vi "Open Waveform File Plot.vi"(8 "error in (no error)":errorcluster, 10 "File Path Control":path, 11 "Measure Controller in":refnum<class "Measure Controller.lvclass">) -> (0 "error out":errorcluster, 3 "Measure Controller out":refnum<class "Measure Controller.lvclass">)   [LabVIEW 2015, in "Measure Controller.lvclass"]
uses:
  Measure Controller.lvclass
  Plots/Waveform Plot/Waveform Plot.lvclass
  Plots/Plot/Plot.lvclass/Plot.ctl
  <vilib>/ActorFramework/Message Enqueuer/Message Enqueuer.lvclass/Message Enqueuer.ctl
  Plots/Plot/Write File-group-channel.vi
  <vilib>/ActorFramework/Message Enqueuer/Enqueue.vi
  <vilib>/ActorFramework/Message Priority Queue/Priority Enqueue.vi
  Measure Object Messages/Open Front Panel Msg/Open Front Panel Msg.lvclass
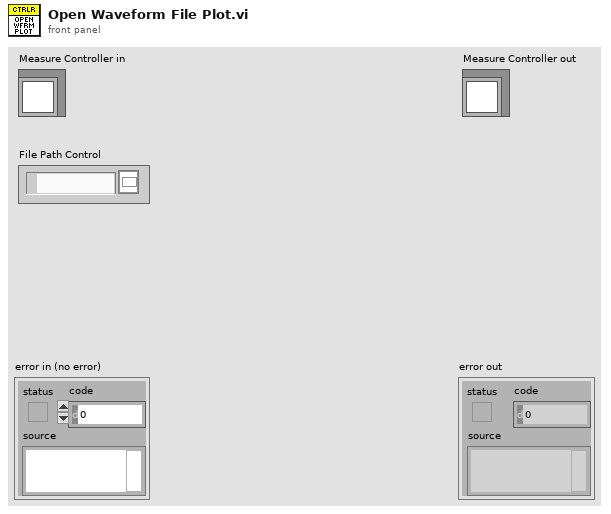
[diagram p1: front panel]
types:
  T1 = cluster{"File Path Control":path, "Group":string, "Channel":string, "Abbreviated":string}
  T2 = cluster{"File Path Control":path, "Group":string, "Channel":string, "Abbreviated":string}[]
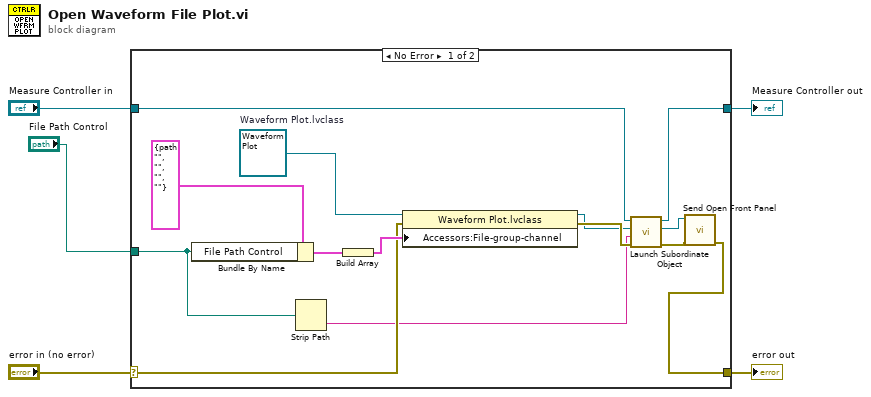
[diagram p0: block diagram]
diagram:
  n1 = case shown="No Error" "error in (no error)" {
    selector: "error in (no error)" -> [w15 w21]
    tunnel: [w6 w21] -> w4
    tunnel: [w13 w20] -> w2
    tunnel: "Measure Controller in" -> [w14 w20]
    tunnel: "File Path Control" -> [w10 _]
    frame No Error {
      w19 = refnum<class "Waveform Plot.lvclass"> refnum  # Waveform Plot.lvclass
      n2 = Bundle By Name(cluster=T1 {"File Path Control"=path "", "Group"="", "Channel"="", "Abbreviated"=""} ("Cluster"), "File Path Control"=w10) -> (w17:T1)
      n3 = Strip Path(path=w10) -> (name=w9:string)  [unwired: 1 out]
      n4 = Build Array(w17) -> (w16:T2)
      n5 = property class="Waveform Plot.lvclass"(reference=w19, error in=w15, "Accessors:File-group-channel"=w16) -> (reference out=w11:refnum<class "Waveform Plot.lvclass">, error out=w12:errorcluster)
      n6 = call-dynamic "Launch Subordinate Object.vi"("error in (no error)"=w12, "Name"=w9, "Subordinate Object"=w11, "Measure Object in"=w14) -> ("error out"=w7:errorcluster, "Nested Actor's Enqueuer"=w8:refnum<class "Message Enqueuer.lvclass">, "Measure Object out"=w13:refnum<class "Measure Controller.lvclass">)  [unwired: 5 in]
      n7 = call "Send Open Front Panel.vi"("error in (no error)"=w7, "Message Enqueuer"=w8) -> ("error out"=w6:errorcluster)  [unwired: 8 in, 1 out]
    }
    frame Error {
    }
  }
  "error out" <- w4
  "Measure Controller out" <- w2
